vi "GPRS自动测试软件.vi"() -> ()   [LabVIEW 2015]
panel:
  out "开始测试时间":timestamp
  in  "设备编号":i32
  in  "测试说明界面参数":T1
  out "测试项目队列":refnum<queue>
  in  "切换卡片界面名称":T2=enum."初始化配置"
  out "指令参数":T3={"测试指令1"={"写参数一"="+TXYBJT GPSQ", "写参数二"="+TXYBJT GPID", "读取版本号"="+TXYBJT GPST", "读取参数一"="+TXYBJT GPCH1", "读取参数二"="+TXYBJT GPCH2", "上电联网"="+TXYBJT GPSM", "指令下线"="+TXYBJT GPSS", "指示灯"=[]}, "测试指令2"={"读取信号强度"="+TXYBJT GPSQ", "读取SIM信息"="+TXYBJT GPID", "读取位置信息"="+TXYBJT GPST", "切换中心参数一"="+TXYBJT GPCH1", "切换中心参数二"="+TXYBJT GPCH2", "强制短信一"="+TXYBJT GPSM", "强制短信二"="+TXYBJT GPSS", "指示灯"=[]}, "等待时间"=[], "校验字符"=[], "GPRS参数"={"GPRS参数一"="", "GPRS参数二"=""}}
  out "状态机状态":T7
  out "当前串口号":refnum<visa-resource-name>
  in  "当前消息":string
  in  "error in":errorcluster caption="error out"
  out "error out":errorcluster
  in  "切换卡片":T8(tab)
  in  "配置串口":bool
  in  "模块参数":bool
  in  "查看配置":bool
  in  "测试网络":bool
  in  "检索模块":bool
  in  "未定义 2":bool
  in  "开始测试":bool
  in  "未定义 4":bool
  in  "测试项目":bool
  out "初始化提示":string
  in  "阿里云网络信息":T9={"IP地址"="192.168.1.2", "端口号"=502}
  out "SMS":bool
  out "UDP":bool
  in  "GPRS参数":enum32{"中心参数一", "中心参数二"}(tab)
  out "GPRS参数1":T10={"IP地址"="192.168.1.1", "工作模式"=48, "连接协议"=48, "本机号码"="13806871122", "短信监控中心号码1"="13800577500", "监听时间"=0, "心跳间隔"=0, "重启时间(分)"=0, "C/S关系"=48, "DNS域名"="", "APN接入点"="", "报头使能"=48, "波特率"=45060, "短信目标号码1 "="", "短信目标号码2"="", "短信监控中心号码2"="", "信号检测使能"=48, "控制方式"=48, "端口号"=5070, "连接方式"=48} {"连接方式" items=["固定IP"=48, "域名解析"=49]; "控制方式" items=["软件控制"=48, "EN控制"=49]; "信号检测使能" items=["不检测"=48, "检测"=49]; "波特率" items=["1200"=51, "2400"=52, "4800"=48, "9600"=49, "19200"=50]; "报头使能" items=["上传"=48, "不上传"=49]; "C/S关系" items=["客服端"=48, "服务端"=49]; "连接协议" items=["TCP协议"=48, "UDP协议"=49]; "工作模式" items=["GPRS模式"=48, "短信模式"=49]}
  out "GPRS参数2":T10={"IP地址"="192.168.1.1", "工作模式"=48, "连接协议"=48, "本机号码"="13806871122", "短信监控中心号码1"="13800577500", "监听时间"=0, "心跳间隔"=0, "重启时间(分)"=0, "C/S关系"=48, "DNS域名"="", "APN接入点"="", "报头使能"=48, "波特率"=45060, "短信目标号码1 "="", "短信目标号码2"="", "短信监控中心号码2"="", "信号检测使能"=48, "控制方式"=48, "端口号"=5070, "连接方式"=48} {"连接方式" items=["固定IP"=48, "域名解析"=49]; "控制方式" items=["软件控制"=48, "EN控制"=49]; "信号检测使能" items=["不检测"=48, "检测"=49]; "波特率" items=["1200"=51, "2400"=52, "4800"=48, "9600"=49, "19200"=50]; "报头使能" items=["上传"=48, "不上传"=49]; "C/S关系" items=["客服端"=48, "服务端"=49]; "连接协议" items=["TCP协议"=48, "UDP协议"=49]; "工作模式" items=["GPRS模式"=48, "短信模式"=49]}
  out "SMS":bool
  out "UDP":bool
  out "TCP":bool
  in  "软件串口参数":T11={"COM号"="COM2", "波特率"=4800, "数据比特"=8, "奇偶"=enum."None", "停止位"=10, "流控制"=0} {"流控制" items=["无"=0, "XON/XOFF"=1, "RTS/CTS"=2, "DTR/DSR"=4]; "停止位" items=["1.0"=10, "1.5"=15, "2.0"=20]; "数据比特" min=5 max=8 step=1; "波特率" items=["75"=75, "110"=110, "134"=134, "150"=150, "300"=300, "600"=600, "1200"=1200, "1800"=1800, "2400"=2400, "4800"=4800, "7200"=7200, "9600"=9600, "14400"=14400, "19200"=19200, "28800"=28800, "38400"=38400, "56000"=56000, "57600"=57600, "115200"=115200, "128000"=128000, "230400"=230400]}
  in  "本地网络信息":T9={"IP地址"="192.168.1.2", "端口号"=502}
  out "TCP":bool
  out "数据测试结果":T12={"读取信号强度"="1", "读取SIM信息"="8", "读取位置信息"="74", "切换中心参数一"="250", "切换中心参数二"="680", "强制短信一"="1024", "强制短信二"="1500", "1"=FALSE, "2"=FALSE, "3"=FALSE, "4"=FALSE, "testw2-udp"=FALSE, "testw0-sms\n 2"=FALSE, "tech-tcp"=FALSE, "tech-udp"=FALSE, "tech-sms"=FALSE, "testr0-tcp\n"=FALSE, "testr0-udp\n"=FALSE, "testr0-sms\n"=FALSE, "testr2-tcp"=FALSE, "testr2-udp"=FALSE, "testr2-sms"=FALSE, "gpon-tcp"=FALSE, "gpon-udp\n"=FALSE, "gpon-sms\n"=FALSE, "gpof-tcp\n"=FALSE, "gpof-udp"=FALSE, "gpof-sms"=FALSE}
  in  "数据测试测试数据":string
  in  "最低工作温度":dbl
  in  "EN=1，待机电流":dbl
  in  "EN=0，待机电流":dbl
  in  "导出按钮":bool
  in  "报告路径":bool
  out "Table":string[][](table) caption="预览"
  out "当前时间":string
  # "TER   TCP  UDP  SMS"
  # "TER   TCP  UDP  SMS"
  # "PCB\n1、添加串口监听\n2、设计手持设备，\n2.1、获取网页数据\n2.2、设置模块参数\n2.3、低功耗\n2.4、通过串口通讯\n3、阿里云创建网页\n爬虫数据"
  # "波特率测试"
  # "1200->4800"
  # "tech"
  # "安排：\n1、重新画板子\n2、添加的单片机\n3、检测电流\n4、485通讯-温度\n5、采用数码管显示\n6、指示灯测试"
  # "域名测试"
  # "测试条件："
  # "重启时间\t30分钟\n心跳间隔\t60s\n监听时间\t0\nEN控制\t是(必须)\n测试时间\t1小时"
  # "开始时间"
  # "结束时间"
  # "允许误差"
  # "是否通过"
  # "TCP"
  # "UDP"
  # "SMS"
  # "现场升级"
  # "远程升级"
  # "测试参数\t\t步骤\t\t时间\t结果\n当前协议\t切换协议\t\t\t\t\nTCP\tTCP\t相同的协议，请确保切换的参数不一样\t\t\t\nTCP\tUDP\t\t\t\t\nTCP\tGSM\t\t\t\t\nUDP\tTCP\t\t\t\t\nUDP\tUDP\t\t\t\t\nUDP\tGSM\t\t\t\t\nGSM\tTCP\t\t\t\t\nGSM\tUDP\t\t\t\t\nGSM\tGSM"
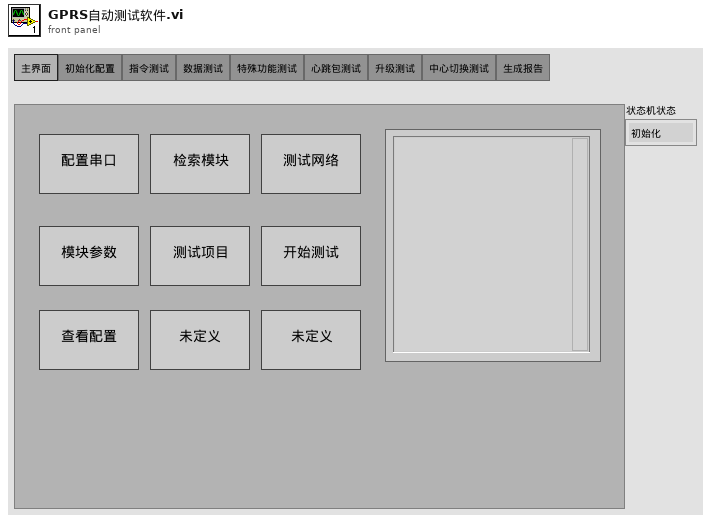
[diagram p1: front panel]
types:
  T1 = typedef "测试说明界面参数.ctl" = cluster{"程序版本":string, "测试软件":string, "说明书版本":string, "测试模块编号":string, "测试内容":string, "问题项目数量":string, "测试人员":string, "报告时间":string, "测试总耗时":string}
  T2 = typedef "切换卡片界面名称.ctl" = enum32{"主界面", "初始化配置", "指令测试", "数据测试", "特殊功能测试", "心跳包测试", "升级测试", "中心切换测试", "生成报告"}
  T3 = typedef "初始化测试指令.ctl" = cluster{"测试指令1":T4, "测试指令2":T5, "等待时间":u32[], "校验字符":string[], "GPRS参数":T6}
  T4 = typedef "指令参数1.ctl" = cluster{"写参数一":string, "写参数二":string, "读取版本号":string, "读取参数一":string, "读取参数二":string, "上电联网":string, "指令下线":string, "指示灯":bool[][]}
  T5 = typedef "指令参数2.ctl" = cluster{"读取信号强度":string, "读取SIM信息":string, "读取位置信息":string, "切换中心参数一":string, "切换中心参数二":string, "强制短信一":string, "强制短信二":string, "指示灯":bool[][]}
  T6 = typedef "GPRS参数.ctl" = cluster{"GPRS参数一":string, "GPRS参数二":string}
  T7 = typedef "状态机状态.ctl" = enum16{"初始化", "等待按键", "串口操作", "检索模块", "网络测试", "测试项目", "模块参数配置", "指令测试", "数据测试", "特殊功能测试", "心跳包测试", "升级测试", "中心切换测试", "计算测试耗时", "生成报告", "提示消息", "退出"}
  T8 = enum32{"主界面", "初始化配置", "指令测试", "数据测试", "特殊功能测试", "心跳包测试", "升级测试", "中心切换测试", "生成报告"}
  T9 = typedef "网络参数.ctl" = cluster{"IP地址":string, "端口号":u16}
  T10 = typedef "GPRS参数DW02.ctl" = cluster{"IP地址":string, "工作模式":u16, "连接协议":u16, "本机号码":string, "短信监控中心号码1":string, "监听时间":u16, "心跳间隔":u16, "重启时间(分)":u16, "C/S关系":u16, "DNS域名":string, "APN接入点":string, "报头使能":u16, "波特率":u16, "短信目标号码1 ":string, "短信目标号码2":string, "短信监控中心号码2":string, "信号检测使能":u16, "控制方式":u16, "端口号":u16, "连接方式":u16}
  T11 = typedef "Serial - Settings.ctl" = cluster{"COM号":refnum<visa-resource-name>, "波特率":u32, "数据比特":u16, "奇偶":enum16{"None", "Odd", "Even", "Mark", "Space"}, "停止位":u16, "流控制":u16}
  T12 = cluster{"读取信号强度":string, "读取SIM信息":string, "读取位置信息":string, "切换中心参数一":string, "切换中心参数二":string, "强制短信一":string, "强制短信二":string, "1":bool, "2":bool, "3":bool, "4":bool, "testw2-udp":bool, "testw0-sms\n 2":bool, "tech-tcp":bool, "tech-udp":bool, "tech-sms":bool, "testr0-tcp\n":bool, "testr0-udp\n":bool, "testr0-sms\n":bool, "testr2-tcp":bool, "testr2-udp":bool, "testr2-sms":bool, "gpon-tcp":bool, "gpon-udp\n":bool, "gpon-sms\n":bool, "gpof-tcp\n":bool, "gpof-udp":bool, "gpof-sms":bool}
  T13 = cluster{"FALSE":bool, "属性节点禁止显示":enum8{"Enabled", "Disabled", "Disabled and Grayed Out"}, "空字符串":string}
  T14 = typedef "初始化测试环境.ctl" = cluster{"串口设置":T11, "网络参数":T9, "测试选项":T15}
  T15 = typedef "测试项目.ctl" = cluster{"指令测试":bool, "特殊功能测试":bool, "数据测试":bool, "心跳包测试":bool, "升级测试":bool, "中心切换测试":bool, "生成报告":bool}
  T16 = enum32{"invalid app kind", "Development System", "Run Time System", "Student Edition", "Embedded LabVIEW", "Evaluation", "Custom"}
  T17 = typedef "检索模块.ctl" = cluster{"发送指令":string, "等待时间（毫秒）":u32, "响应数据":string, "波特率":T18}
  T18 = typedef "波特率.ctl" = u32[]
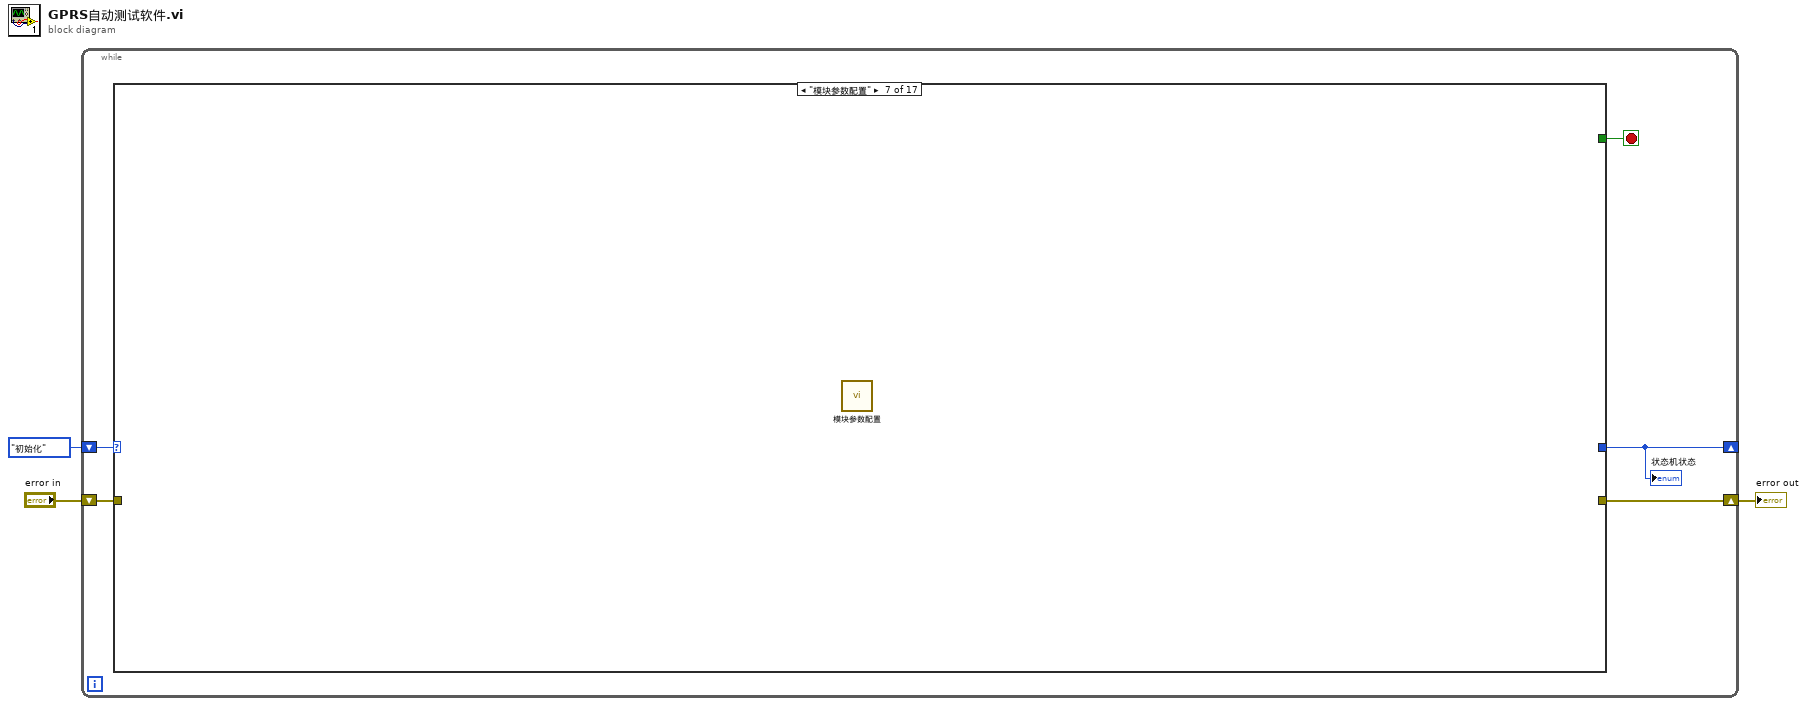
[diagram p0: block diagram]
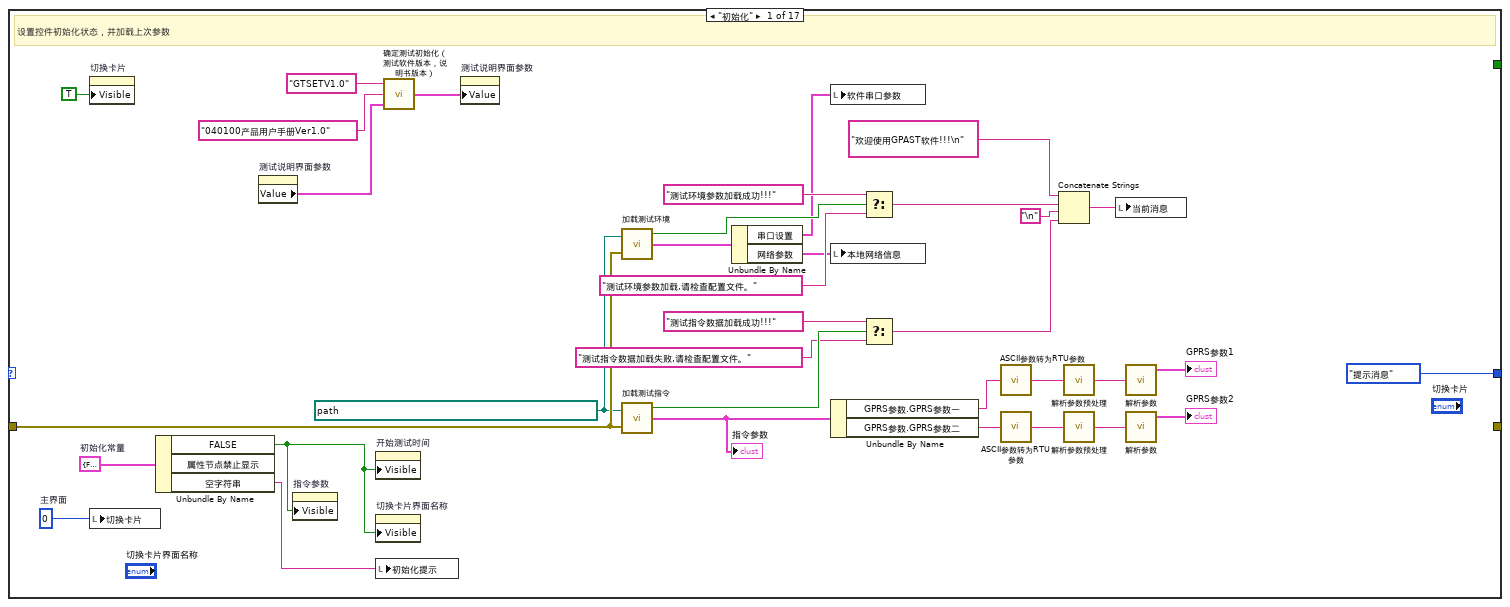
[diagram p2: hidden frame]
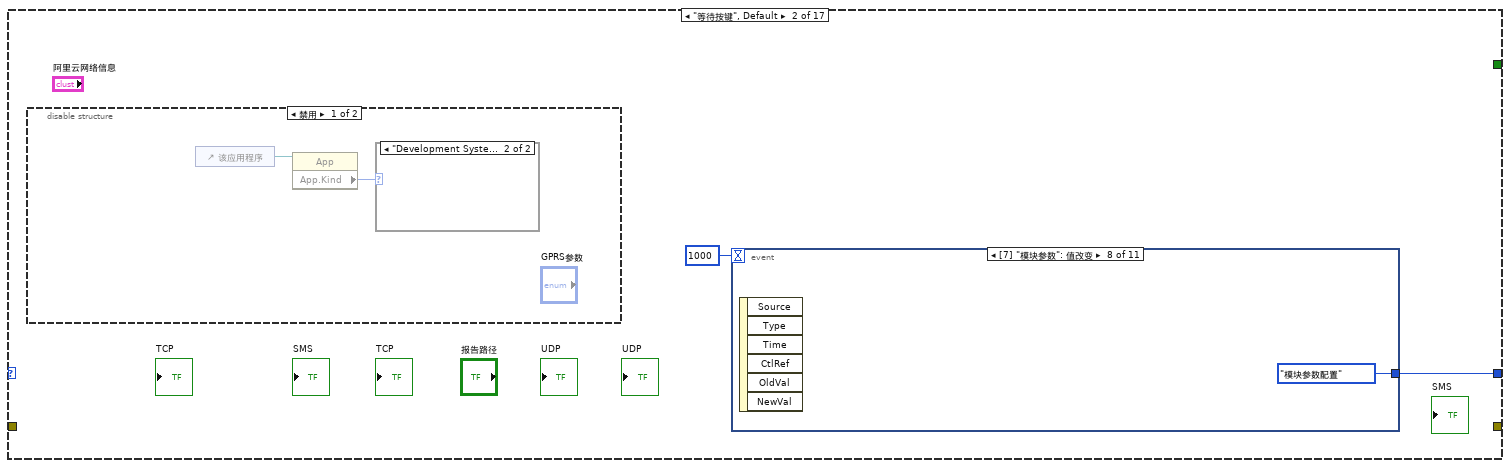
[diagram p3: hidden frame]
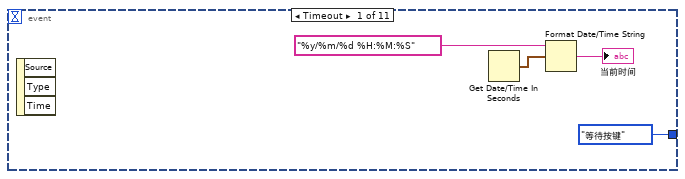
[diagram p6: hidden frame]
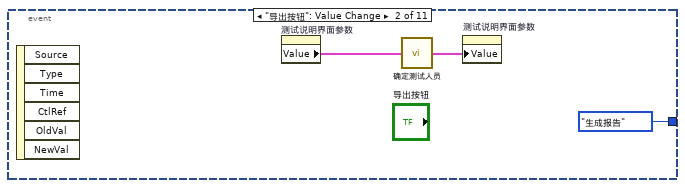
[diagram p7: hidden frame]
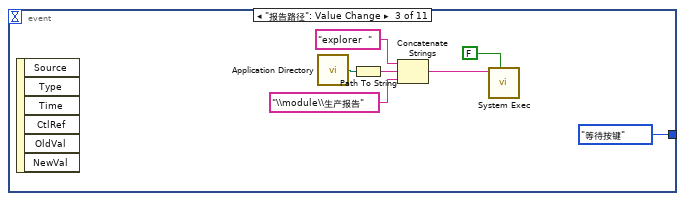
[diagram p8: hidden frame]
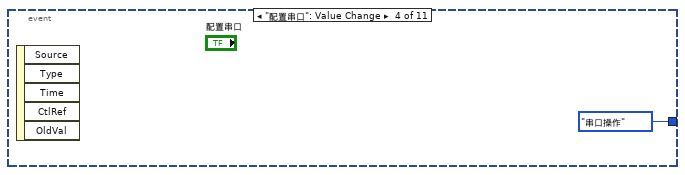
[diagram p9: hidden frame]
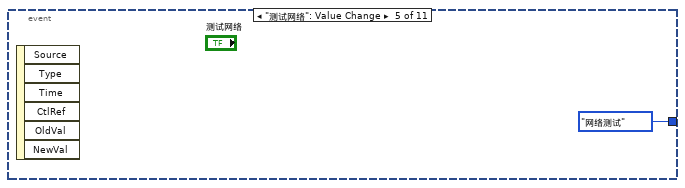
[diagram p10: hidden frame]
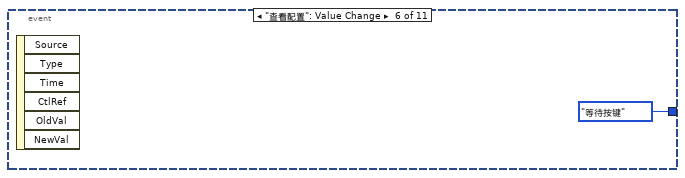
[diagram p11: hidden frame]
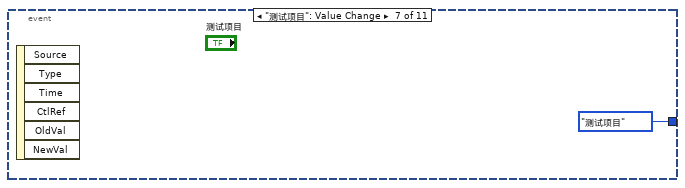
[diagram p12: hidden frame]
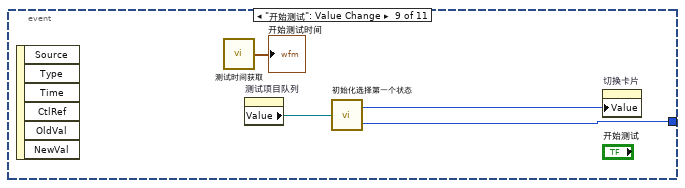
[diagram p13: hidden frame]
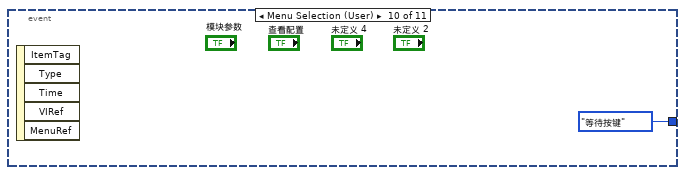
[diagram p14: hidden frame]
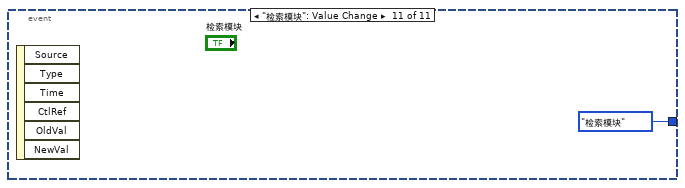
[diagram p15: hidden frame]
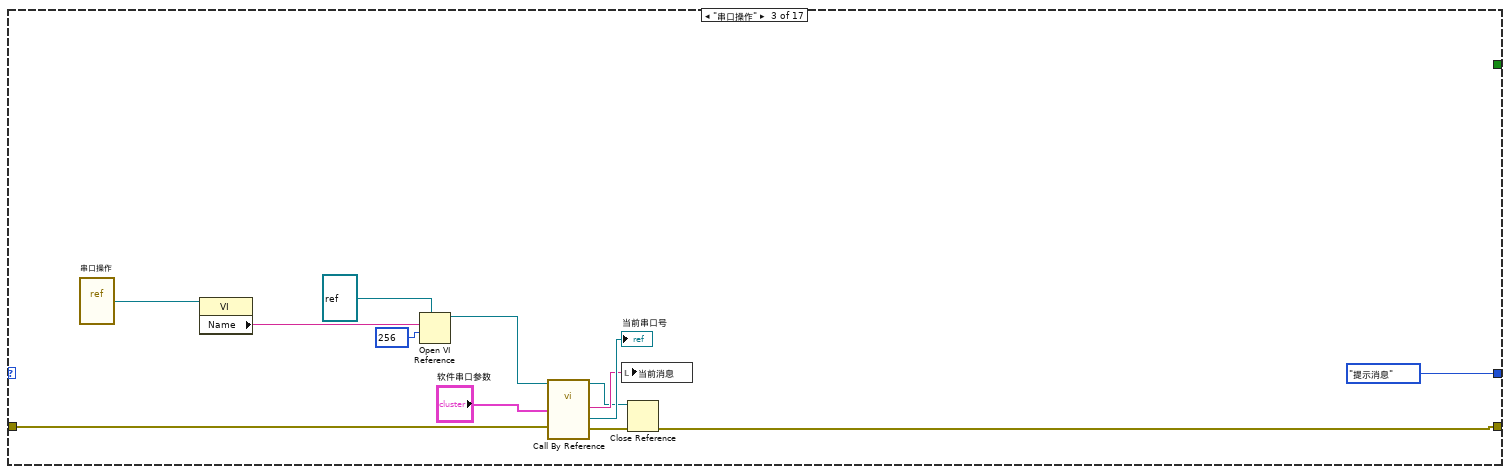
[diagram p16: hidden frame]
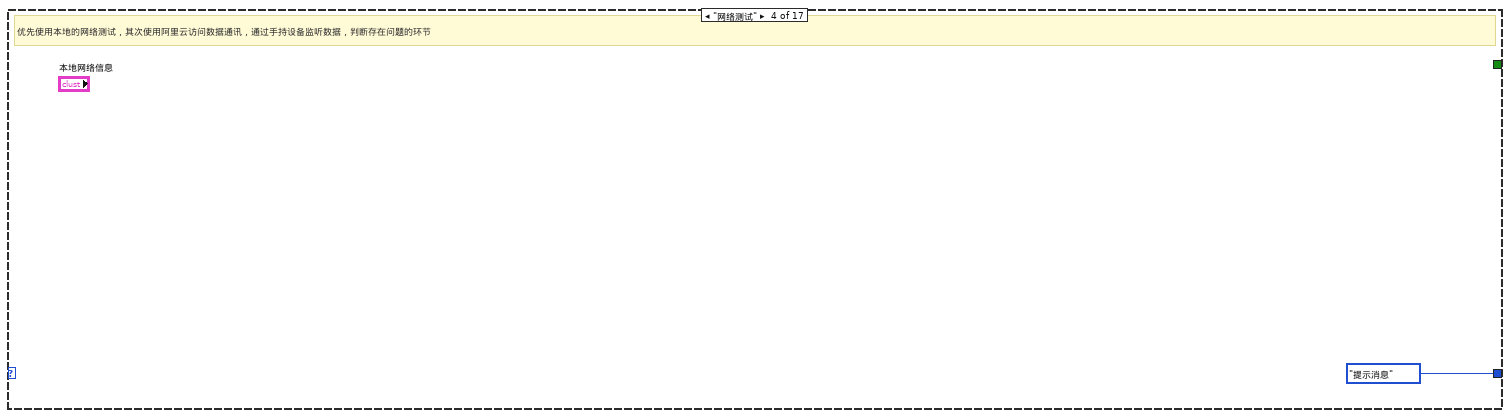
[diagram p17: hidden frame]
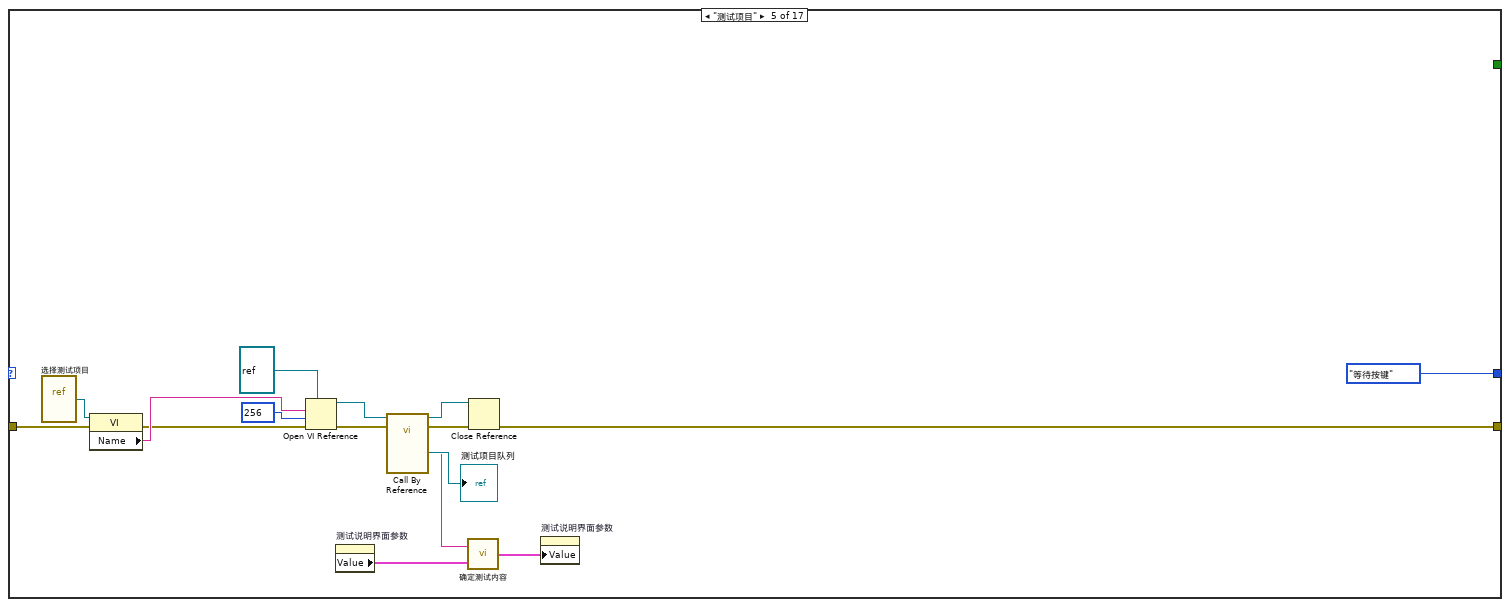
[diagram p18: hidden frame]
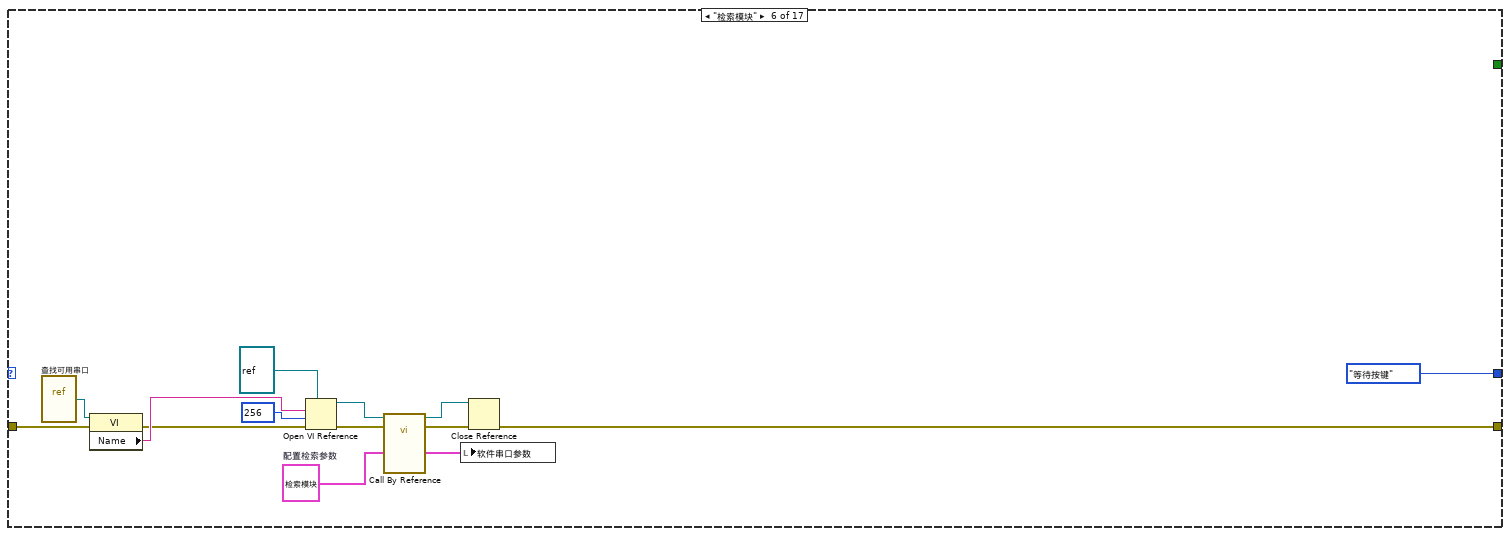
[diagram p19: hidden frame]
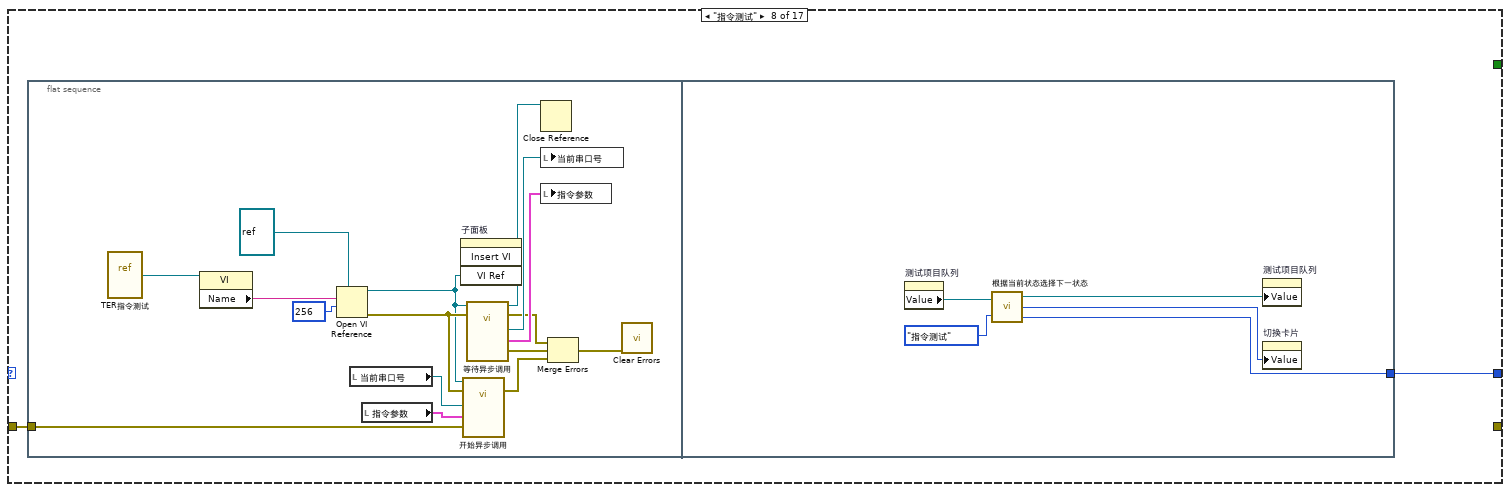
[diagram p20: hidden frame]
diagram:
  n1 = while {
    shift-right: [w8] -> w2
    shift-left: "error in" -> [w6]
    shift-right: [w5] -> _
    shift-left: 状态机状态."初始化" -> [w7]
    stop <- w4 stop-if-true
    n2 = case shown="\"模块参数配置\"" w7 {
      tunnel: [_ _ w75 _ w91 w104 _ _ _ _ _ _ _ _ w182 w193 _] -> w8
      tunnel: w6 -> [w39 _ w79 _ w96 w105 _ w118 _ _ _ _ _ _ w188 w193 _]
      tunnel: [状态机状态."提示消息" w45 状态机状态."提示消息" 状态机状态."提示消息" 状态机状态."等待按键" 状态机状态."等待按键" _ w117 w140 w147 w157 w163 w169 状态机状态."等待按键" 状态机状态."等待按键" 状态机状态."等待按键" 状态机状态."退出"] -> w5
      tunnel: [_ _ _ _ _ _ _ _ _ _ _ _ _ _ _ _ TRUE] -> w4
      frame "初始化" {
        w25 = 0  # 主界面
        w11 = path "F:/Project/GPRS测试/GPRS测试上位机/GPATS.ini" ("configuration file path")
        w36 = T13 {"FALSE"=FALSE, "属性节点禁止显示"=enum."Disabled and Grayed Out", "空字符串"=""}  # 初始化常量
        # "设置控件初始化状态，并加载上次参数"
        n3 = property on="切换卡片" class="TabCtl (严格)"("Visible"=TRUE ("可见")) -> ()  [unwired: 2 in, 2 out]
        n4 = local write "切换卡片"(w25) -> ()
        n5 = Unbundle By Name(w36) -> ("FALSE"=w19:bool, "空字符串"=w35:string)  [unwired: 1 out]
        n6 = property on="测试说明界面参数" class="Clust (严格)"() -> ("Value"=w21:T1)  [unwired: 2 in, 2 out]
        n7 = property on="指令参数" class="Clust (严格)"("Visible"=w19) -> ()  [unwired: 2 in, 2 out]
        n8 = property on="开始测试时间" class="AbsTime (严格)"("Visible"=w19) -> ()  [unwired: 2 in, 2 out]
        n9 = property on="切换卡片界面名称" class="Enum (严格)"("Visible"=w19) -> ()  [unwired: 2 in, 2 out]
        n10 = local write "初始化提示"(w35) -> ()
        n11 = call "确定测试初始化（测试软件版本，说明书版本）.vi"("测试说明界面参数输入"=w21, "说明书版本"="040100产品用户手册Ver1.0", "测试软件"="GTSETV1.0") -> ("测试说明界面参数输出"=w20:T1)
        n12 = property on="测试说明界面参数" class="Clust (严格)"("Value"=w20) -> ()  [unwired: 2 in, 2 out]
        n13 = call "加载测试环境.vi"("输入ini文件地址"=w11, "error in (no error)"=w39) -> ("加载成功?"=w34:bool, "测试环境参数"=w31:T14)  [unwired: 1 out]
        n14 = call "加载测试指令.vi"("输入ini文件地址"=w11, "error in (no error)"=w39) -> ("加载成功?"=w28:bool, "指令参数"=w18:T3)  [unwired: 1 out]
        "指令参数" <- w18
        n15 = Unbundle By Name(w31) -> ("串口设置"=w30:T11, "网络参数"=w29:T9)
        n16 = local write "软件串口参数"(w30) -> ()
        n17 = local write "本地网络信息"(w29) -> ()
        n18 = Unbundle By Name(w18) -> ("GPRS参数.GPRS参数一"=w17:string, "GPRS参数.GPRS参数二"=w14:string)
        n19 = Select(t="测试环境参数加载成功!!!" ("f"), s=w34, f="测试环境参数加载,请检查配置文件。") -> (s? t:f=w42:string)
        n20 = Select(t="测试指令数据加载成功!!!" ("f"), s=w28, f="测试指令数据加载失败,请检查配置文件。") -> (s? t:f=w38:string)
        n21 = call "ASCII参数转为RTU参数.vi"("ASCII参数"=w17) -> ("RTU参数"=w13:string)
        n22 = call "ASCII参数转为RTU参数.vi"("ASCII参数"=w14) -> ("RTU参数"=w15:string)
        n23 = Concatenate Strings("欢迎使用GPAST软件!!!\n" ("初始化提示"), w42, "\n" ("字符串"), w38) -> (w40:string)
        n24 = call "解析参数预处理.vi"("待解析参数内容"=w13) -> ("字符串"=w12:string)
        n25 = call "解析参数预处理.vi"("待解析参数内容"=w15) -> ("字符串"=w16:string)
        n26 = local write "当前消息"(w40) -> ()
        n27 = call "解析参数.vi"("输入字符串"=w12) -> ("GPRS参数（TXJT）"=→"GPRS参数1":T10)  [unwired: 2 out]
        n28 = call "解析参数.vi"("输入字符串"=w16) -> ("GPRS参数（TXJT）"=→"GPRS参数2":T10)  [unwired: 2 out]
      }
      frame "等待按键", Default {
        n29 = disable-structure shown="禁用" {
          frame Disabled {
            n30 = control-ref of="该应用程序"() -> (w46:refnum<vi>)
            n31 = property class="App"(reference=w46) -> ("App.Kind"=w47:T16)  [unwired: 1 in, 2 out]
            n32 = case shown="\"Development System\"" w47 {
              frame "invalid app kind", Default {
              }
              frame "Development System" {
              }
            }
          }
          frame Enabled {
          }
        }
        n33 = event shown="[7] \"模块参数\": 值改变" {
          selector: _ -> [_ _ _ _ _ _ _ _ _ _ _]
          dyn-events: _ -> [_ _ _ _ _ _ _ _ _ _ _]
          timeout: 1000 -> [_ _ _ _ _ _ _ _ _ _ _]
          tunnel: [状态机状态."等待按键" 状态机状态."生成报告" 状态机状态."等待按键" 状态机状态."串口操作" 状态机状态."网络测试" 状态机状态."等待按键" 状态机状态."测试项目" 状态机状态."模块参数配置" w69 状态机状态."等待按键" 状态机状态."检索模块"] -> w45
          event Timeout {
            n34 = event-data() -> ()  [unwired: 1 in, 3 out]
            n35 = Get Date/Time In Seconds() -> (seconds since 1Jan1904=w50:timestamp)
            n36 = Format Date/Time String(time format string (%c)="%y/%m/%d %H:%M:%S" ("时间格式字符串(%c)"), seconds (now)=w50) -> (date/time string=→"当前时间":string)  [unwired: 1 in]
          }
          event "导出按钮": Value Change {
            n37 = event-data() -> ()  [unwired: 1 in, 6 out]
            n38 = property on="测试说明界面参数" class="Clust (严格)"() -> ("Value"=w52:T1)  [unwired: 2 in, 2 out]
            n39 = call "确定测试人员.vi"("测试说明界面参数输入"=w52) -> ("测试说明界面参数输出"=w53:T1)
            n40 = property on="测试说明界面参数" class="Clust (严格)"("Value"=w53) -> ()  [unwired: 2 in, 2 out]
          }
          event "报告路径": Value Change {
            n41 = event-data() -> ()  [unwired: 1 in, 6 out]
            n42 = call <vilib>:"Application Directory.vi"() -> ("Application Directory"=w58:path)
            n43 = Path To String(path=w58) -> (string=w60:string)
            n44 = Concatenate Strings("explorer  " ("字符串"), w60, "\\module\\生产报告" ("名称或相对路径")) -> (w56:string)
            n45 = call <vilib>:"System Exec.vi"("wait until completion? (T)"=FALSE, "command line"=w56) -> ()  [unwired: 6 in, 4 out]
          }
          event "配置串口": Value Change {
            n46 = event-data() -> ()  [unwired: 1 in, 5 out]
          }
          event "测试网络": Value Change {
            n47 = event-data() -> ()  [unwired: 1 in, 6 out]
          }
          event "查看配置": Value Change {
            n48 = event-data() -> ()  [unwired: 1 in, 6 out]
          }
          event "测试项目": Value Change {
            n49 = event-data() -> ()  [unwired: 1 in, 6 out]
          }
          event "模块参数": Value Change {
            n50 = event-data() -> ()  [unwired: 1 in, 6 out]
          }
          event "开始测试": Value Change {
            n51 = event-data() -> ()  [unwired: 1 in, 6 out]
            n52 = call "测试时间获取.vi"() -> ("time stamp"=→"开始测试时间":timestamp)  [unwired: 1 in]
            n53 = property on="测试项目队列" class="TypRef (严格)"() -> ("Value"=w67:refnum<queue>)  [unwired: 2 in, 2 out]
            n54 = call "初始化选择第一个状态.vi"("测试项目队列输入"=w67) -> ("切换卡片"=w70:T8, "当前状态"=w69:T7)
            n55 = property on="切换卡片" class="TabCtl (严格)"("Value"=w70) -> ()  [unwired: 2 in, 2 out]
          }
          event Menu Selection (User) {
            n56 = event-data() -> ()  [unwired: 1 in, 5 out]
          }
          event "检索模块": Value Change {
            n57 = event-data() -> ()  [unwired: 1 in, 6 out]
          }
        }
      }
      frame "串口操作" {
        n58 = vi-ref "串口操作.vi"() -> (w84:refnum<vi>)
        n59 = property class="VI"(reference=w84) -> ("Name"=w83:string)  [unwired: 1 in, 2 out]
        n60 = Open VI Reference(type specifier VI Refnum (for type only)=refnum<vi> refnum ("类型说明符VI引用句柄（仅用于类型）"), vi path=w83, options=256 ("选项")) -> (vi reference=w81:refnum<vi>)  [unwired: 3 in, 1 out]
        n61 = call-by-ref "?"(reference=w81, "串口设置"="软件串口参数", "错误输入（无错误）"=w79) -> (reference out=w74:refnum<vi>, "输出最后的消息"=w77:string, "当前串口号"=→"当前串口号":refnum<visa-resource-name>, "错误输出"=w76:errorcluster)  [unwired: 1 in, 1 out]
        n62 = local write "当前消息"(w77) -> ()
        n63 = Close Reference(reference=w74, error in (no error)=w76) -> (error out=w75:errorcluster)
      }
      frame "网络测试" {
        # "优先使用本地的网络测试，其次使用阿里云访问数据通讯，通过手持设备监听数据，判断存在问题的环节"
      }
      frame "测试项目" {
        n64 = vi-ref "选择测试项目.vi"() -> (w100:refnum<vi>)
        n65 = property class="VI"(reference=w100, error in=w96) -> (error out=w98:errorcluster, "Name"=w101:string)  [unwired: 1 out]
        n66 = Open VI Reference(type specifier VI Refnum (for type only)=refnum<vi> refnum ("类型说明符VI引用句柄（仅用于类型）"), vi path=w101, options=256 ("选项"), error in (no error)=w98) -> (vi reference=w95:refnum<vi>, error out=w94:errorcluster)  [unwired: 2 in]
        n67 = property on="测试说明界面参数" class="Clust (严格)"() -> ("Value"=w87:T1)  [unwired: 2 in, 2 out]
        n68 = call-by-ref "?"(reference=w95, error in=w94) -> (reference out=w93:refnum<vi>, error out=w92:errorcluster, "报告测试内容"=w88:string, "queue out"=→"测试项目队列":refnum<queue>)
        n69 = call "确定测试内容.vi"("测试说明界面参数输入"=w87, "测试内容"=w88) -> ("测试说明界面参数输出"=w89:T1)
        n70 = Close Reference(reference=w93, error in (no error)=w92) -> (error out=w91:errorcluster)
        n71 = property on="测试说明界面参数" class="Clust (严格)"("Value"=w89) -> ()  [unwired: 2 in, 2 out]
      }
      frame "检索模块" {
        w110 = T17 {"发送指令"="+TXYBJT TECH", "等待时间（毫秒）"=500, "响应数据"="DTU Software,VER", "波特率"=[1200, 2400, 4800, 9600, 19200]}  # 配置检索参数
        n72 = vi-ref "查找可用串口.vi"() -> (w115:refnum<vi>)
        n73 = property class="VI"(reference=w115, error in=w105) -> (error out=w106:errorcluster, "Name"=w114:string)  [unwired: 1 out]
        n74 = Open VI Reference(type specifier VI Refnum (for type only)=refnum<vi> refnum ("类型说明符VI引用句柄（仅用于类型）"), vi path=w114, options=256 ("选项"), error in (no error)=w106) -> (vi reference=w112:refnum<vi>, error out=w107:errorcluster)  [unwired: 2 in]
        n75 = call-by-ref "?"(reference=w112, error in=w107, "配置检索参数"=w110) -> (reference out=w109:refnum<vi>, error out=w108:errorcluster, "已检索串口参数"=w111:T11)
        n76 = local write "软件串口参数"(w111) -> ()
        n77 = Close Reference(reference=w109, error in (no error)=w108) -> (error out=w104:errorcluster)
      }
      frame "模块参数配置" {
        n78 = call "模块参数配置.vi"() -> ()  [unwired: 12 in]
      }
      frame "指令测试" {
        n79 = flat-sequence {
          tunnel: w118 -> [w131]
          tunnel: [w138] -> w117
          frame #0 {
            n80 = vi-ref "TER指令测试.vi"() -> (w129:refnum<vi>)
            n81 = property class="VI"(reference=w129) -> ("Name"=w128:string)  [unwired: 1 in, 2 out]
            n82 = Open VI Reference(type specifier VI Refnum (for type only)=refnum<vi> refnum ("类型说明符VI引用句柄（仅用于类型）"), vi path=w128, options=256 ("选项")) -> (vi reference=w124:refnum<vi>, error out=w130:errorcluster)  [unwired: 3 in]
            n83 = local read "当前串口号"() -> (w132:refnum<visa-resource-name>)
            n84 = local read "指令参数"() -> (w133:T3)
            n85 = invoke on="子面板" class="SubPnl" method="Insert VI"("VI Ref"=w124) -> ()  [unwired: 3 in, 4 out]
            n86 = call-by-ref "开始异步调用"(reference=w124, error in=w130, "错误输入（无错误）"=w131, "指令参数输入"=w133, "VISA引用句柄输入"=w132) -> (error out=w120:errorcluster)  [unwired: 4 out]
            n87 = call-by-ref "等待异步调用"(reference=w124, error in=w130) -> (reference out=w125:refnum<vi>, error out=w122:errorcluster, "错误输出"=w121:errorcluster, "指令参数输出"=w127:T3, "VISA引用句柄输出"=w126:refnum<visa-resource-name>)  [unwired: 3 in]
            n88 = Close Reference(reference=w125) -> ()  [unwired: 1 in, 1 out]
            n89 = local write "当前串口号"(w126) -> ()
            n90 = local write "指令参数"(w127) -> ()
            n91 = Merge Errors(w122, w121, w120) -> (w119:errorcluster)
            n92 = call <vilib>:"Clear Errors.vi"("error in (no error)"=w119) -> ()  [unwired: 5 in, 2 out]
          }
          frame #1 {
            n93 = property on="测试项目队列" class="TypRef (严格)"() -> ("Value"=w136:refnum<queue>)  [unwired: 2 in, 2 out]
            n94 = call "根据当前状态选择下一状态.vi"("测试项目队列输入"=w136, "当前状态"=状态机状态."指令测试") -> ("测试项目队列输出"=w135:refnum<queue>, "切换卡片界面名称"=w137:T2, "下一状态"=w138:T7)
            n95 = property on="测试项目队列" class="TypRef (严格)"("Value"=w135) -> ()  [unwired: 2 in, 2 out]
            n96 = property on="切换卡片" class="TabCtl (严格)"("Value"=w137) -> ()  [unwired: 2 in, 2 out]
          }
        }
      }
      frame "数据测试" {
        n97 = flat-sequence {
          tunnel: [w146] -> w140
          frame #0 {
            n98 = Wait (ms)(milliseconds to wait=u32 3000 ("等待时间（毫秒）")) -> ()  [unwired: 1 out]
          }
          frame #1 {
            n99 = property on="测试项目队列" class="TypRef (严格)"() -> ("Value"=w143:refnum<queue>)  [unwired: 2 in, 2 out]
            n100 = call "根据当前状态选择下一状态.vi"("测试项目队列输入"=w143, "当前状态"=状态机状态."数据测试") -> ("测试项目队列输出"=w142:refnum<queue>, "切换卡片界面名称"=w144:T2, "下一状态"=w146:T7)
            n101 = local write "切换卡片"(w144) -> ()
            n102 = property on="测试项目队列" class="TypRef (严格)"("Value"=w142) -> ()  [unwired: 2 in, 2 out]
          }
        }
      }
      frame "特殊功能测试" {
        n103 = flat-sequence {
          tunnel: [w151] -> w147
          frame #0 {
            n104 = Wait (ms)(milliseconds to wait=u32 3000 ("等待时间（毫秒）")) -> ()  [unwired: 1 out]
          }
          frame #1 {
            n105 = property on="测试项目队列" class="TypRef (严格)"() -> ("Value"=w150:refnum<queue>)  [unwired: 2 in, 2 out]
            n106 = call "根据当前状态选择下一状态.vi"("测试项目队列输入"=w150, "当前状态"=状态机状态."特殊功能测试") -> ("测试项目队列输出"=w149:refnum<queue>, "切换卡片界面名称"=w152:T2, "下一状态"=w151:T7)
            n107 = property on="切换卡片" class="TabCtl (严格)"("Value"=w152) -> ()  [unwired: 2 in, 2 out]
            n108 = property on="测试项目队列" class="TypRef (严格)"("Value"=w149) -> ()  [unwired: 2 in, 2 out]
          }
        }
      }
      frame "心跳包测试" {
        n109 = Wait (ms)(milliseconds to wait=u32 3000 ("等待时间（毫秒）")) -> ()  [unwired: 1 out]
        n110 = property on="测试项目队列" class="TypRef (严格)"() -> ("Value"=w155:refnum<queue>)  [unwired: 2 in, 2 out]
        n111 = call "根据当前状态选择下一状态.vi"("测试项目队列输入"=w155, "当前状态"=状态机状态."心跳包测试") -> ("测试项目队列输出"=w154:refnum<queue>, "切换卡片界面名称"=w158:T2, "下一状态"=w157:T7)
        n112 = property on="切换卡片" class="TabCtl (严格)"("Value"=w158) -> ()  [unwired: 2 in, 2 out]
        n113 = property on="测试项目队列" class="TypRef (严格)"("Value"=w154) -> ()  [unwired: 2 in, 2 out]
      }
      frame "升级测试" {
        n114 = Wait (ms)(milliseconds to wait=u32 3000 ("等待时间（毫秒）")) -> ()  [unwired: 1 out]
        n115 = property on="测试项目队列" class="TypRef (严格)"() -> ("Value"=w161:refnum<queue>)  [unwired: 2 in, 2 out]
        n116 = call "根据当前状态选择下一状态.vi"("测试项目队列输入"=w161, "当前状态"=状态机状态."升级测试") -> ("测试项目队列输出"=w160:refnum<queue>, "切换卡片界面名称"=w164:T2, "下一状态"=w163:T7)
        n117 = property on="切换卡片" class="TabCtl (严格)"("Value"=w164) -> ()  [unwired: 2 in, 2 out]
        n118 = property on="测试项目队列" class="TypRef (严格)"("Value"=w160) -> ()  [unwired: 2 in, 2 out]
      }
      frame "中心切换测试" {
        n119 = Wait (ms)(milliseconds to wait=u32 3000 ("等待时间（毫秒）")) -> ()  [unwired: 1 out]
        n120 = property on="测试项目队列" class="TypRef (严格)"() -> ("Value"=w167:refnum<queue>)  [unwired: 2 in, 2 out]
        n121 = call "根据当前状态选择下一状态.vi"("测试项目队列输入"=w167, "当前状态"=状态机状态."中心切换测试") -> ("测试项目队列输出"=w166:refnum<queue>, "切换卡片界面名称"=w170:T2, "下一状态"=w169:T7)
        n122 = property on="切换卡片" class="TabCtl (严格)"("Value"=w170) -> ()  [unwired: 2 in, 2 out]
        n123 = property on="测试项目队列" class="TypRef (严格)"("Value"=w166) -> ()  [unwired: 2 in, 2 out]
      }
      frame "计算测试耗时" {
        n124 = call "测试时间获取.vi"() -> ("time stamp"=w180:timestamp)  [unwired: 1 in]
        n125 = property on="开始测试时间" class="AbsTime (严格)"() -> ("Value"=w176:timestamp)  [unwired: 2 in, 2 out]
        n126 = Subtract(x=w180, y=w176) -> (x-y=w179:dbl)
        n127 = Number To Decimal String(number=w179) -> (decimal integer string=w174:string)  [unwired: 1 in]
        n128 = property on="测试说明界面参数" class="Clust (严格)"() -> ("Value"=w178:T1)  [unwired: 2 in, 2 out]
        n129 = Concatenate Strings(w174, "s" ("字符串")) -> (w172:string)
        n130 = call "确定测试总耗时.vi"("测试说明界面参数输入"=w178, "测试总耗时"=w172) -> ("测试说明界面参数输出"=w177:T1)
        n131 = property on="测试说明界面参数" class="Clust (严格)"("Value"=w177) -> ()  [unwired: 2 in, 2 out]
      }
      frame "生成报告" {
        n132 = property on="测试说明界面参数" class="Clust (严格)" props=["Value"]() -> ()  [unwired: 2 in, 3 out]
        n133 = property on="测试项目队列" class="TypRef (严格)"() -> ("Value"=w189:refnum<queue>)  [unwired: 2 in, 2 out]
        n134 = Release Queue(queue=w189, error in (no error)=w188) -> (error out=w183:errorcluster)  [unwired: 1 in, 2 out]
        n135 = Increment(x="设备编号") -> (x+1=w186:i32)
        n136 = call "确定测试模块编号.vi"("测试说明界面参数输入"="测试说明界面参数", "设备编号"=w186) -> ("测试说明界面参数输出"=w184:T1)
        n137 = call "确定测试报告时间.vi"("测试说明界面参数输入"=w184) -> ("测试说明界面参数输出"=w181:T1)
        n138 = call "生成测试说明界面.vi"("错误输入（无错误）"=w183, "测试说明界面参数"=w181) -> ("错误输出"=w182:errorcluster)
      }
      frame "提示消息" {
        n139 = Empty String/Path?(string/path="当前消息") -> (empty?=w192:bool)
        n140 = case shown="真" w192 {
          tunnel: "当前消息" -> [w197 _]
          frame False {
            w200 = "\r\n" ("字符串")
            n141 = Get Date/Time In Seconds() -> (seconds since 1Jan1904=w202:timestamp)
            n142 = local write "当前消息"("") -> ()
            n143 = local read "初始化提示"() -> (w196:string)
            n144 = property on="初始化提示" class="Str"("Text.Scroll Position"=inf) -> ()  [unwired: 2 in, 2 out]
            n145 = Get Date/Time String(seconds (now)=w202) -> (date string=w201:string, time string=w203:string)  [unwired: 2 in]
            n146 = Concatenate Strings(w196, w201, w203, w200, w197, w200) -> (→"初始化提示":string)
          }
          frame True {
          }
        }
      }
      frame "退出" {
        n147 = local read "当前串口号"() -> (w205:refnum<visa-resource-name>)
        n148 = VISA Close(VISA resource name=w205) -> (error out=w204:errorcluster)  [unwired: 1 in]
        n149 = call <vilib>:"Clear Errors.vi"("error in (no error)"=w204) -> ()  [unwired: 5 in, 2 out]
      }
    }
    "状态机状态" <- w5
  }
  "error out" <- w2
